vi "FTW-XML-Destroy.vi"(0 "XML Node":refnum<k20>, 11 "error in":errorcluster) -> (15 "error out":errorcluster)   [LabVIEW 2012]
panel:
  # "Inputs"
  # "Outputs"
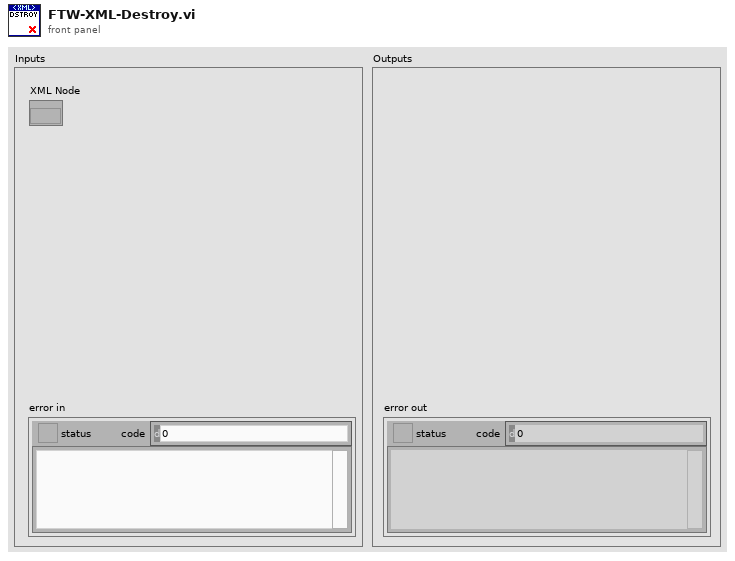
[diagram p1: front panel]
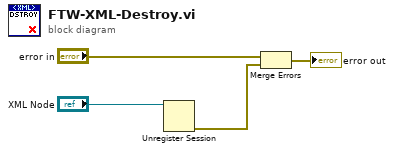
[diagram p0: block diagram]
diagram:
  n1 = Unregister Session(11:"XML Node") -> (0:w1:errorcluster)  [unwired: 1 in]
  n2 = Merge Errors("error in", w1) -> (→"error out":errorcluster)
